vi "color config.vi"(9 "max":dbl, 10 "autoscale":bool, 11 "color 1":T1) -> (2 "max":dbl, 3 "Array":cluster{dbl, u32}[](array[cluster]))   [LabVIEW 2024]
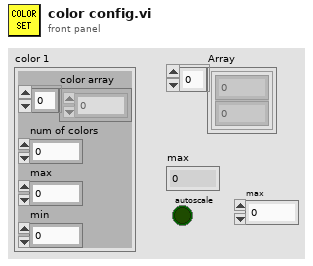
[diagram p1: front panel]
types:
  T1 = cluster{"color array":u32[], "num of colors":i32, "max":dbl, "min":dbl}
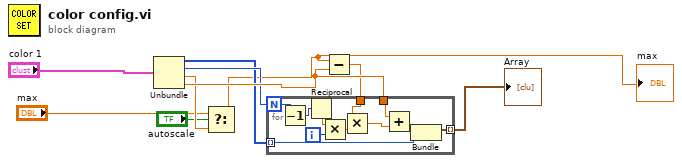
[diagram p0: block diagram]
diagram:
  n1 = Unbundle("color 1") -> ("color array"=w7:u32[], "num of colors"=w8:i32, "max"=w9:dbl, "min"=w10:dbl)
  n2 = Select(t="max", s="autoscale", f=w9) -> (s? t:f=w3:dbl)
  "max" <- w3
  n3 = Subtract(x=w3, y=w10) -> (x-y=w4:dbl)
  n4 = for {
    N: w8 -> [w15]
    tunnel: w4 -> [w19]
    tunnel: [w17] -> w5 mode=indexing
    tunnel: w7 -> [w16] mode=indexing
    tunnel: w10 -> [w11]
    i -> [w21]
    n5 = Decrement(x=w15) -> (x-1=w14:i32)
    n6 = Reciprocal(x=w14) -> (1/x=w13:dbl)
    n7 = Multiply(x=w13, y=w21) -> (x*y=w20:dbl)
    n8 = Multiply(x=w19, y=w20) -> (x*y=w18:dbl)
    n9 = Add(x=w11, y=w18) -> (x+y=w12:dbl)
    n10 = Bundle(w12, w16) -> (w17:cluster{dbl, u32})  [unwired: 1 in]
  }
  "Array" <- w5
